vi "Reject Status.vi"() -> ()   [LabVIEW 2021]
uses:
  Controls/Reject.ctl
panel:
  out "Reject Status":T1
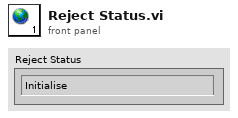
[diagram p1: front panel]
types:
  T1 = typedef "Reject.ctl" = enum16{"Initialise", "CYL Fwd", "Wait for Delay", "CYL Rear", "Done", "Error"}
diagram:
